vi "Resample Waveform (continuous, t0 DBL).vi"(0 "waveform in":waveform(dbl), 1 "reset":bool, 5 "dt":dbl=1.0 format="%.2p", 7 "t0":dbl=-inf format="%.2p", 9 "interpolation mode":u16(ring)=1 items=["coerce", "linear", "spline", "FIR filter"], 11 "error in (no error)":errorcluster, 12 "FIR filter specifications":T1={"alias rejection (dB)"=120.0, "normalized bandwidth"=0.4536} {"normalized bandwidth" format="%.4f"; "alias rejection (dB)" format="%.2f"}) -> (4 "resampled waveform out":waveform(dbl), 8 "next t0":dbl format="%.2p", 10 "used t0":dbl format="%.2p", 14 "t0 adjusted warning":bool, 15 "error out":errorcluster)   [LabVIEW 2020, in "NI_MAPro.lvlib"]
doc: "Resamples an input waveform according to the user-defined values for <B>t0</B> and <B>dt</B>. Wire data to the <B>waveform in</B> input to determine the polymorphic instance to use or manually select the instance."
uses:
  NI_MAPro.lvlib
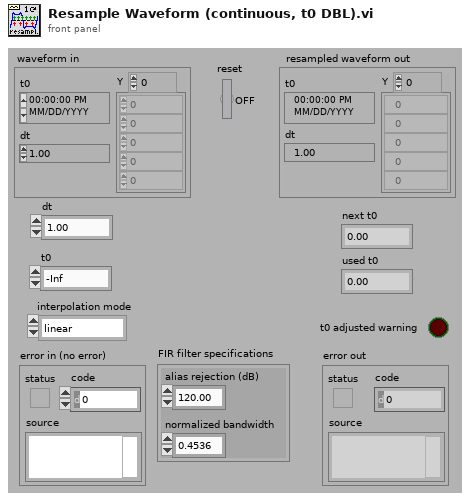
[diagram p1: front panel]
types:
  T1 = cluster{"alias rejection (dB)":dbl, "normalized bandwidth":dbl}
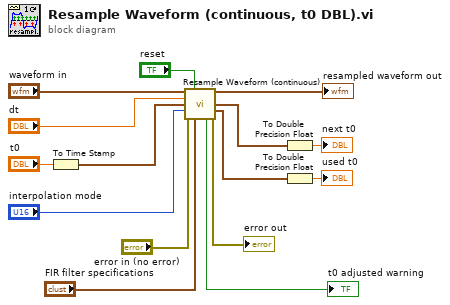
[diagram p0: block diagram]
diagram:
  n1 = To Time Stamp(1:"t0") -> (0:w12:timestamp)
  n2 = call "Resample Waveform (continuous).vi"("waveform in"="waveform in", "reset"="reset", "dt"="dt", "t0"=w12, "interpolation mode"="interpolation mode", "error in (no error)"="error in (no error)", "FIR filter specifications"="FIR filter specifications") -> ("resampled waveform out"=→"resampled waveform out":waveform(dbl), "next t0"=w10:timestamp, "used t0"=w8:timestamp, "t0 adjusted warning"=→"t0 adjusted warning":bool, "error out"=→"error out":errorcluster)  [unwired: 4 in]
  n3 = To Double Precision Float(number=w10) -> (double precision float=→"next t0":dbl)
  n4 = To Double Precision Float(number=w8) -> (double precision float=→"used t0":dbl)
